vi "InitSelfCheck.vi"() -> ()   [LabVIEW 2014]
uses:
  <vilib>/Instr/_visa.llb/VISA Configure Serial Port (Instr).vi
  <vilib>/addons/database/Connection.llb/DB Tools Open Connec (String).vi
  <vilib>/addons/database/Connection.llb/Conn Execute.vi
  <vilib>/addons/database/Recordset.llb/Rec Fetch Recordset Data (R).vi
  <vilib>/addons/database/Recordset.llb/Rec Destroy - Connection.vi
  <vilib>/addons/database/_DB Variant To Data/Database Variant To Data.xnode
  <vilib>/addons/database/NI_Database_API.lvlib
panel:
  out "错误输出 2":errorcluster caption="错误输出"
  out "String":string
  out "Slide":u8(slide) scale=0.0..50.0
  out "Current Status":string
  # "自检中...请稍候\n\n\n--"
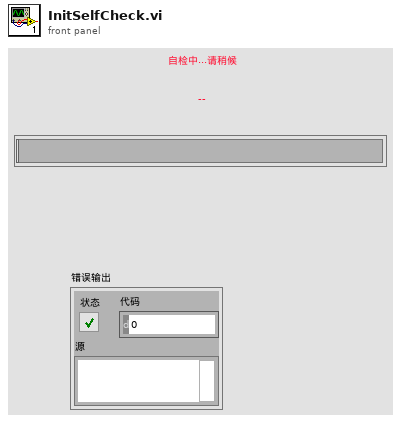
[diagram p1: front panel]
types:
  T1 = typedef "NI_Database_API.lvlib/Conn ObjectReference.ctl" = refnum<k1>
  T2 = typedef "NI_Database_API.lvlib/Rec ObjectReference.ctl" = refnum<k1>
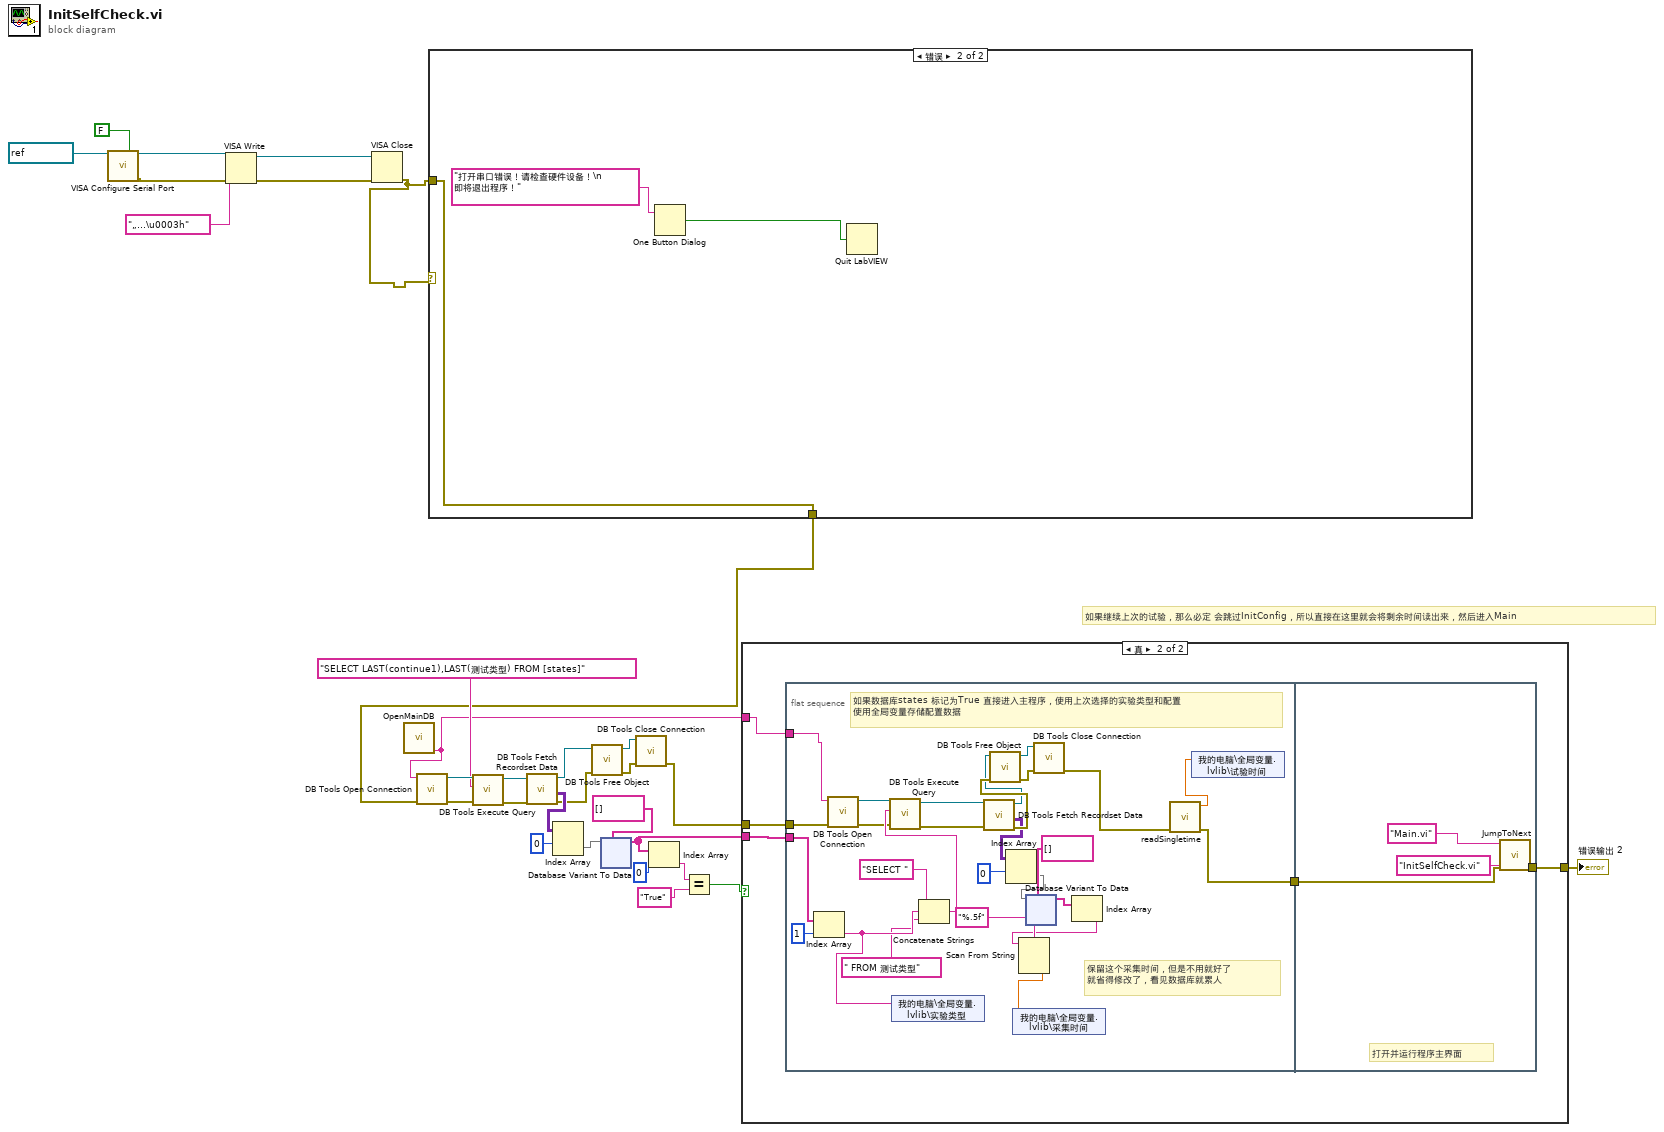
[diagram p0: block diagram]
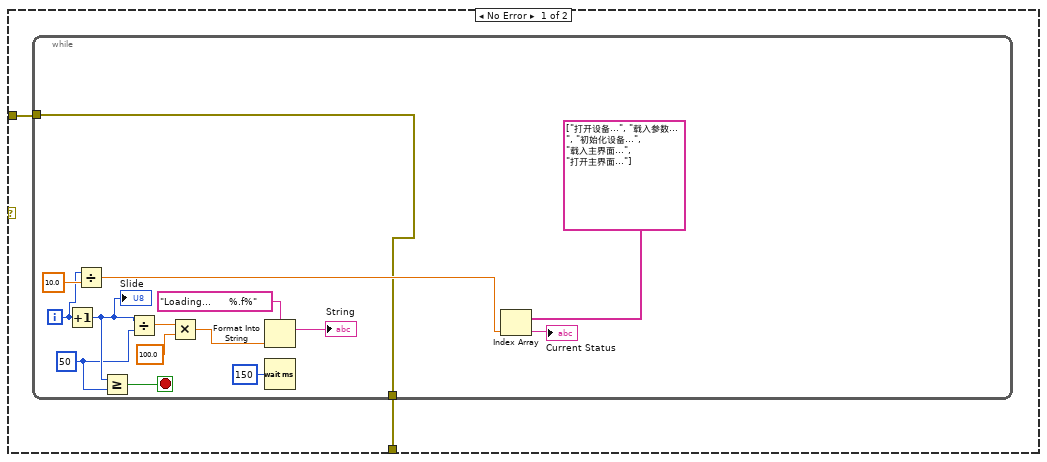
[diagram p2: hidden frame]
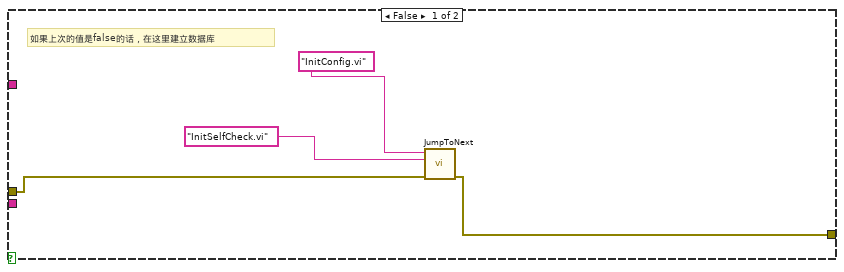
[diagram p3: hidden frame]
diagram:
  # "如果继续上次的试验，那么必定 会跳过InitConfig，所以直接在这里就会将剩余时间读出来，然后进入Main"
  n1 = call-poly "VISA Configure Serial Port"("VISA resource name"=refnum<visa-resource-name> "COM2", "Enable Termination\nChar (T)"=FALSE ("Enable Termination\nChar (T)")) -> ("VISA resource name out"=w6:refnum<visa-resource-name>, "error out"=w5:errorcluster)  [unwired: 12 in]
  n2 = VISA Write(VISA resource name=w6, write buffer="„…\u0003h" ("写入缓冲区"), error in (no error)=w5) -> (VISA resource name out=w7:refnum<visa-resource-name>, error out=w8:errorcluster)  [unwired: 1 out]
  n3 = VISA Close(VISA resource name=w7, error in (no error)=w8) -> (error out=w1:errorcluster)
  n4 = call "OpenMainDB.vi"() -> ("头信息"=w12:string)  [unwired: 11 in]
  n5 = case shown="错误" w1 {
    tunnel: [w32 w48] -> w9
    tunnel: w1 -> [w31 w48]
    frame No Error {
      n6 = while {
        tunnel: [w33] -> w32
        tunnel: w31 -> [w33]
        i -> [w35]
        stop <- w45 stop-if-true
        w42 = 50 ("y")
        n7 = Increment(x=w35) -> (x+1=w44:i32)
        "Slide" <- w44
        n8 = Divide(x=w35, y=10.0) -> (x/y=w34:dbl)
        n9 = Greater Or Equal?(x=w44, y=w42) -> (x >= y?=w45:bool)
        n10 = Divide(x=w44, y=w42) -> (x/y=w43:dbl)
        n11 = Multiply(x=w43, y=100.0) -> (x*y=w40:dbl)
        n12 = Format Into String(format string="Loading...      %.f%", w40) -> (resulting string=→"String":string)  [unwired: 2 in, 1 out]
        n13 = Wait (ms)(milliseconds to wait=u32 150) -> ()  [unwired: 1 out]
        n14 = Index Array(array=string[] ["打开设备...", "载入参数...", "初始化设备...", "载入主界面...", "打开主界面..."], index=w34) -> (element=→"Current Status":string)
      }
    }
    frame Error {
      n15 = One Button Dialog(message="打开串口错误！请检查硬件设备！\n         即将退出程序！") -> (true=w49:bool)  [unwired: 1 in]
      n16 = Quit LabVIEW(quit? (T)=w49) -> ()
    }
  }
  n17 = call-poly <vilib>:"DB Tools Open Connection.vi"("error in (no error)"=w9, "connection information"=w12) -> ("error out"=w30:errorcluster, "connection reference"=w29:T1)  [unwired: 6 in]
  n18 = call-poly <vilib>:"DB Tools Execute Query.vi"("error in (no error)"=w30, "SQL query"="SELECT LAST(continue1),LAST(测试类型) FROM [states]", "connection reference"=w29) -> ("error out"=w26:errorcluster, "recordset reference"=w27:T2)  [unwired: 5 in]
  n19 = call-poly <vilib>:"DB Tools Fetch Recordset Data.vi"("error in (no error)"=w26, "recordset reference"=w27) -> ("error out"=w16:errorcluster, "recordset data"=w25:variant[][], "recordset reference out"=w17:T2)  [unwired: 3 in]
  n20 = Index Array(array=w25, index (row)=0 ("索引 (行)")) -> (element=w23:variant[])  [unwired: 1 in]
  n21 = call-poly <vilib>:"DB Tools Free Object.vi"("error in (no error)"=w16, "recordset reference"=w17) -> ("error out"=w14:errorcluster, "connection reference"=w15:T1)  [unwired: 8 in]
  n22 = xnode "Database Variant To Data"("database variant"=w23, "type"=string[] []) -> ("data"=w13:string[])  [unwired: 1 in, 1 out]
  n23 = call <vilib>:"DB Tools Close Connection.vi"("error in (no error)"=w14, "connection reference"=w15) -> ("error out"=w11:errorcluster)  [unwired: 5 in]
  n24 = Index Array(array=w13, index=0 ("索引")) -> (element=w20:string)
  n25 = Equal?(x=w20, y="True") -> (x = y?=w18:bool)
  n26 = case shown="真" w18 {
    tunnel: w13 -> [_ w58]
    tunnel: w12 -> [_ w59]
    tunnel: w11 -> [w52 w57]
    tunnel: [w51 w55] -> w10
    frame False {
      # "如果上次的值是false的话，在这里建立数据库"
      n27 = call "JumpToNext.vi"("错误输入（无错误）"=w52, "要关闭的VI"="InitSelfCheck.vi", "要打开的VI"="InitConfig.vi") -> ("错误输出"=w51:errorcluster)  [unwired: 8 in]
    }
    frame True {
      n28 = flat-sequence {
        tunnel: w59 -> [w65]
        tunnel: w58 -> [w64]
        tunnel: w57 -> [w63]
        tunnel: [w61] -> w56
        tunnel: w56 -> [w126]
        tunnel: [w125] -> w55
        frame #0 {
          # "保留这个采集时间，但是不用就好了\n就省得修改了，看见数据库就累人"
          # "如果数据库states 标记为True 直接进入主程序，使用上次选择的实验类型和配置\n使用全局变量存储配置数据"
          n29 = Index Array(array=w64, index=1 ("索引")) -> (element=w86:string)
          n30 = call-poly <vilib>:"DB Tools Open Connection.vi"("error in (no error)"=w63, "connection information"=w65) -> ("error out"=w68:errorcluster, "connection reference"=w67:T1)  [unwired: 6 in]
          n31 = shared-variable "我的电脑\\全局变量.lvlib\\实验类型"(w86) -> ()  [unwired: 1 in, 1 out]
          n32 = Concatenate Strings("SELECT ", w86, " FROM 测试类型") -> (w71:string)
          n33 = call-poly <vilib>:"DB Tools Execute Query.vi"("error in (no error)"=w68, "SQL query"=w71, "connection reference"=w67) -> ("error out"=w73:errorcluster, "recordset reference"=w72:T2)  [unwired: 5 in]
          n34 = call-poly <vilib>:"DB Tools Fetch Recordset Data.vi"("error in (no error)"=w73, "recordset reference"=w72) -> ("error out"=w82:errorcluster, "recordset data"=w75:variant[][], "recordset reference out"=w81:T2)  [unwired: 3 in]
          n35 = call-poly <vilib>:"DB Tools Free Object.vi"("error in (no error)"=w82, "recordset reference"=w81) -> ("error out"=w79:errorcluster, "connection reference"=w80:T1)  [unwired: 8 in]
          n36 = Index Array(array=w75, index (row)=0 ("索引 (行)")) -> (element=w76:variant[])  [unwired: 1 in]
          n37 = xnode "Database Variant To Data"("database variant"=w76, "type"=string[] []) -> ("data"=w78:string[])  [unwired: 1 in, 1 out]
          n38 = call <vilib>:"DB Tools Close Connection.vi"("error in (no error)"=w79, "connection reference"=w80) -> ("error out"=w62:errorcluster)  [unwired: 5 in]
          n39 = Index Array(array=w78) -> (element=w83:string)  [unwired: 1 in]
          n40 = Scan From String(format string="%.5f" ("格式字符串"), input string=w83) -> (output 1=w85:dbl)  [unwired: 3 in, 3 out]
          n41 = shared-variable "我的电脑\\全局变量.lvlib\\采集时间"(w85) -> ()  [unwired: 1 in, 1 out]
          n42 = call "readSingletime.vi"("error in (no error)"=w62) -> ("error out"=w61:errorcluster, "试验时间"=w60:dbl)  [unwired: 9 in]
          n43 = shared-variable "我的电脑\\全局变量.lvlib\\试验时间"(w60) -> ()  [unwired: 1 in, 1 out]
        }
        frame #1 {
          # "打开并运行程序主界面"
          n44 = call "JumpToNext.vi"("错误输入（无错误）"=w126, "要关闭的VI"="InitSelfCheck.vi", "要打开的VI"="Main.vi") -> ("错误输出"=w125:errorcluster)  [unwired: 8 in]
        }
      }
    }
  }
  "错误输出 2" <- w10
